vi "RCM Send Start Exiting Request MHLC.vi"(8 "error in (no error)":errorcluster, 10 "Tree RCM Data":T1, 11 "AppMgr in":refnum<class "Application Manager.lvclass">) -> (0 "error out":errorcluster, 3 "AppMgr out":refnum<class "Application Manager.lvclass">)   [LabVIEW 2017, in "Application Manager.lvclass"]
doc: "Send Response Message to start the shutdown routine of the selected Worker"
uses:
  Application Manager.lvclass
  Tree Right Click Menu Data.ctl
  <vilib>/Utility/miscctls.llb/LVPoint32TypeDef.ctl
  Application Manager.lvclass/Application Manager.ctl
  rsp_Send Start Exiting Request.ctl
  Common VIs/DC_UID.ctl
  <vilib>/Utility/error.llb/Error Cluster From Error Code.vi
  <vilib>/ErrorRing/Error Ring.xnode
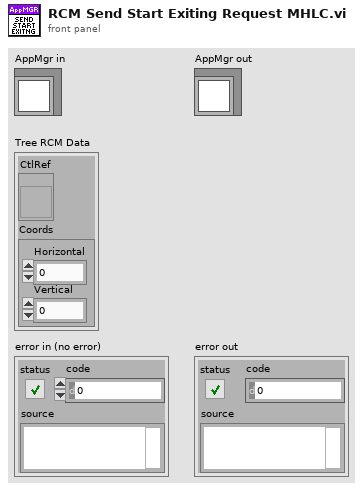
[diagram p1: front panel]
types:
  T1 = typedef "Application Manager.lvclass/Tree Right Click Menu Data.ctl" = cluster{"CtlRef":refnum<vi>, "Coords":T2}
  T2 = typedef "LVPoint32TypeDef.ctl" = cluster{"Horizontal":i32, "Vertical":i32}
  T3 = typedef "DC_UID.ctl" = string
  T4 = typedef "Application Manager.lvclass/Debug Client Data.ctl" = cluster{"DC_UID":T3, "IP Address":string, "Worker Data":T5[], "Connected":bool}
  T5 = typedef "Application Manager.lvclass/Worker Data.ctl" = cluster{"ID":string, "VI Ref":refnum<vi>, "VI Path":path, "CloneID":string, "Type":T6, "Worker Status":string}
  T6 = typedef "Workers.lvlib/Worker.lvclass/Worker Type.ctl" = enum16{"SL", "DL"}
  T7 = typedef "Application Manager.lvclass/rsp_Send Start Exiting Request.ctl" = cluster{"DC_UID":T3, "Worker ID":string}
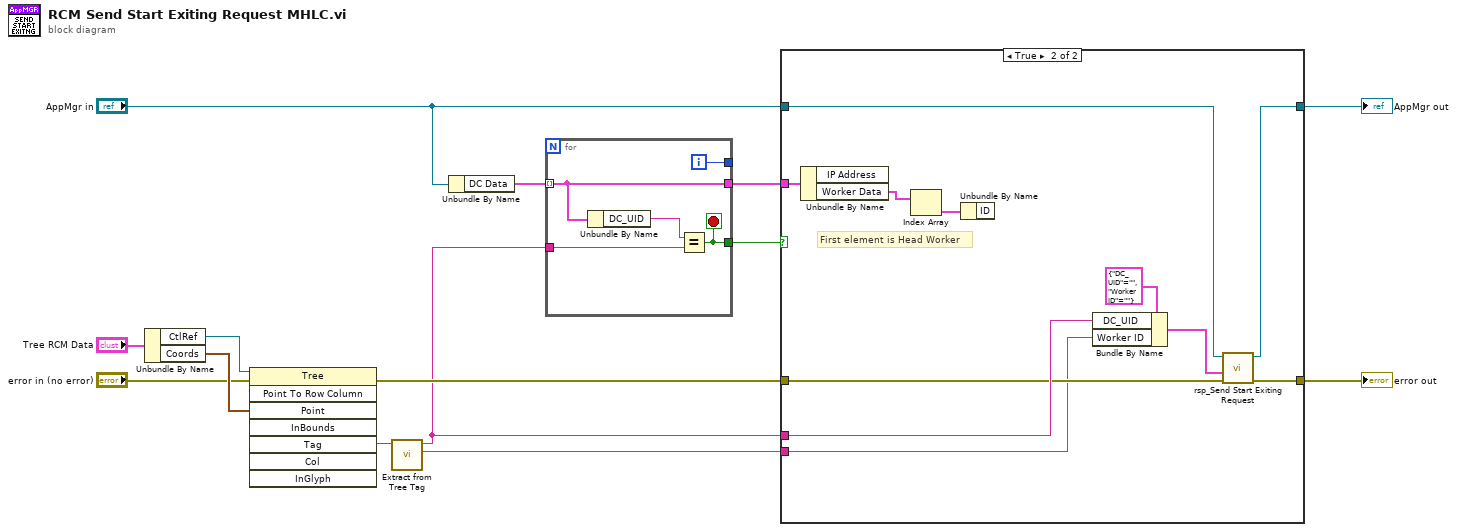
[diagram p0: block diagram]
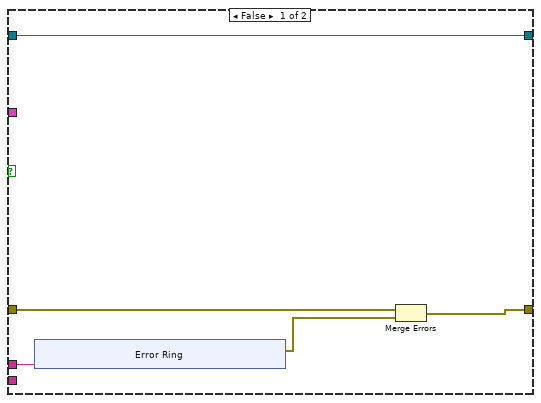
[diagram p2: hidden frame]
diagram:
  n1 = Unbundle By Name("Tree RCM Data") -> ("CtlRef"=w11:refnum<vi>, "Coords"=w10:T2)
  n2 = invoke class="Tree" method="Point To Row Column"(reference=w11, error in="error in (no error)", "Point"=w10) -> (error out=w9:errorcluster, "Tag"=w8:string)  [unwired: 5 in, 6 out]
  n3 = call "Extract from Tree Tag.vi"("Tag"=w8) -> ("WID"=w1:string, "DC_UID"=w7:T3)  [unwired: 9 in]
  n4 = Unbundle By Name("AppMgr in") -> ("DC Data"=w6:T4[])
  n5 = for {
    tunnel: w6 -> [w16] mode=indexing
    tunnel: [w18] -> w4
    tunnel: [w17] -> _
    tunnel: [w16] -> w5
    tunnel: w7 -> [w15]
    i -> [w17]
    stop <- w18 stop-if-true
    n6 = Unbundle By Name(w16) -> ("DC_UID"=w19:T3)
    n7 = Equal?(x=w19, y=w15) -> (x = y?=w18:bool)
  }
  n8 = case shown="True" w4 {
    tunnel: [w23 w35] -> w12
    tunnel: w9 -> [w24 w36]
    tunnel: w7 -> [w21 w37]
    tunnel: w5 -> [_ w42]
    tunnel: "AppMgr in" -> [w20 w39]
    tunnel: [w20 w38] -> w13
    tunnel: w1 -> [_ w32]
    frame False {
      n9 = xnode "Error Ring"("parameter 0"=w21) -> ("error out"=w22:errorcluster)
      n10 = Merge Errors(w24, w22) -> (w23:errorcluster)
    }
    frame True {
      # "First element is Head Worker"
      n11 = Unbundle By Name(w42) -> ("Worker Data"=w34:T5[])  [unwired: 1 out]
      n12 = Index Array(array=w34) -> (element=w33:T5)  [unwired: 1 in]
      n13 = Unbundle By Name(w33) -> ()  [unwired: 1 out]
      n14 = Bundle By Name(cluster=T7 {"DC_UID"="", "Worker ID"=""} ("Data in"), "DC_UID"=w37, "Worker ID"=w32) -> (w41:T7)
      n15 = call "rsp_Send Start Exiting Request.vi"("error in"=w36, "Data in"=w41, "Application Manager in"=w39) -> ("error out"=w35:errorcluster, "dup Application Manager out"=w38:refnum<class "Application Manager.lvclass">)  [unwired: 7 in]
    }
  }
  "AppMgr out" <- w13
  "error out" <- w12
